vi "Handle Array.vi"(7 "Set(f)":bool, 11 "Array Handles":T1(array[cluster])) -> (3 "Array Handles":T1(array[cluster]))   [LabVIEW 2014, in "ScopePlugins.lvlib" / "NIScope.lvclass"]
uses:
  NIScope.lvclass
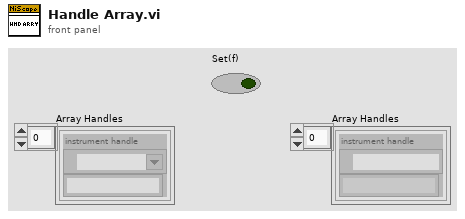
[diagram p1: front panel]
types:
  T1 = cluster{"instrument handle":refnum<k15>, string}[]
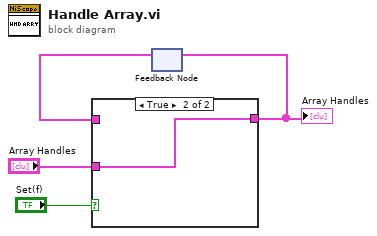
[diagram p0: block diagram]
diagram:
  n1 = feedback #1() -> (w1:T1)  [unwired: 1 in]
  n2 = case shown="True" "Set(f)" {
    tunnel: "Array Handles" -> [_ w6]
    tunnel: [w5 w6] -> w2
    tunnel: w1 -> [w5 _]
    frame False {
    }
    frame True {
    }
  }
  "Array Handles" <- w2
  n3 = feedback-in #1(w2) -> ()
